vi "WaveformChartGraph-Ver2.vi"() -> ()   [LabVIEW 2019]
panel:
  in  "OK Button":bool
  out "Array":dbl[](array[numeric])
  out "Waveform Graph":dbl[](graph)
  out "Waveform Chart":dbl(graph)
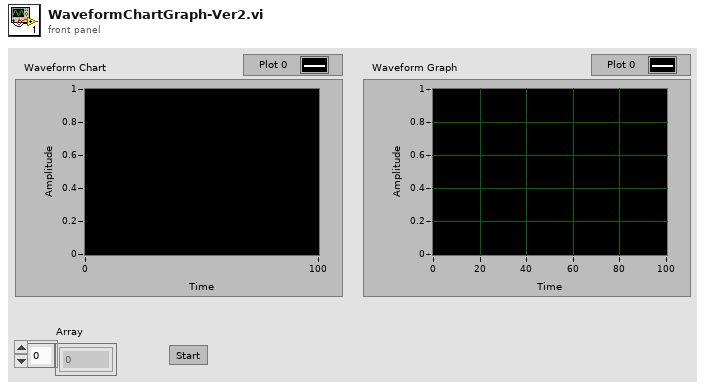
[diagram p1: front panel]
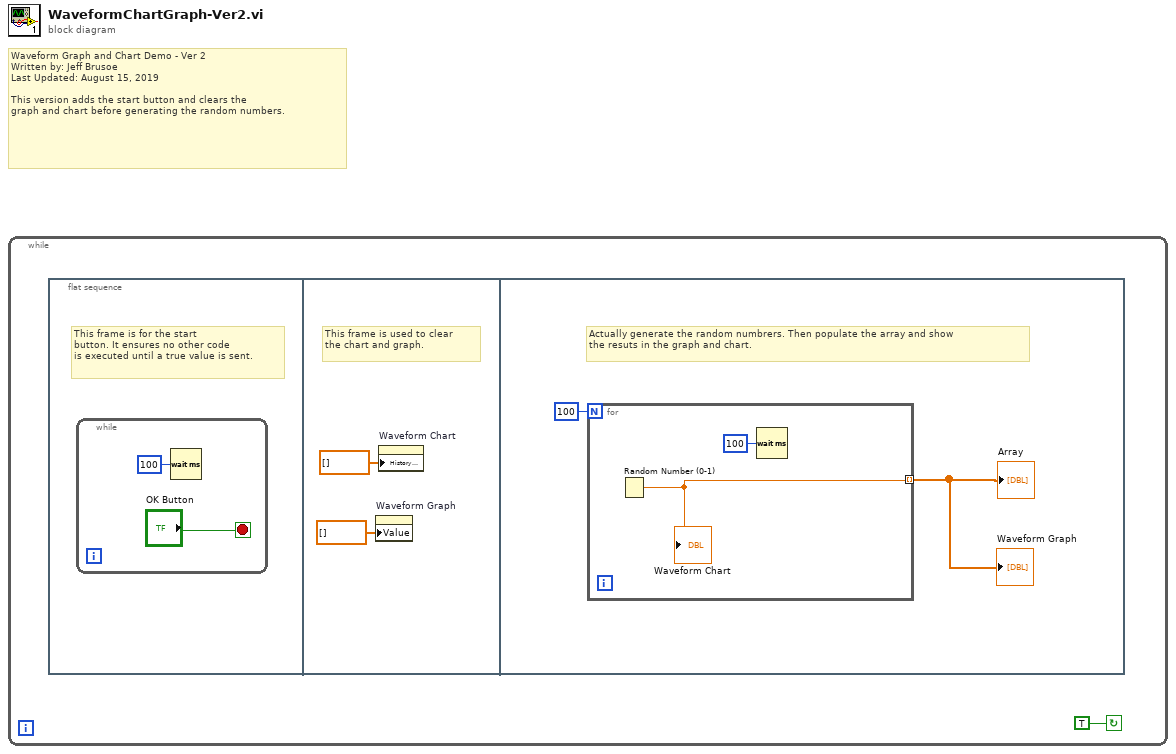
[diagram p0: block diagram]
diagram:
  # "Waveform Graph and Chart Demo - Ver 2\nWritten by: Jeff Brusoe\nLast Updated: August 15, 2019\n\nThis version adds the start button and clears the \ngraph and chart before generating the random numbers."
  n1 = while {
    stop <- TRUE continue-if-true
    n2 = flat-sequence {
      frame #0 {
        # "This frame is for the start\nbutton. It ensures no other code\nis executed until a true value is sent."
        n3 = while {
          stop <- "OK Button" stop-if-true
          n4 = Wait (ms)(milliseconds to wait=u32 100) -> ()  [unwired: 1 out]
        }
      }
      frame #1 {
        # "This frame is used to clear\nthe chart and graph."
        n5 = property on="Waveform Graph" class="WFGraph (strict)"("Value"=dbl[] [] ("Waveform Graph")) -> ()  [unwired: 2 in, 2 out]
        n6 = property on="Waveform Chart" class="WFChart (strict)"("History Data"=dbl[] []) -> ()  [unwired: 2 in, 2 out]
      }
      frame #2 {
        # "Actually generate the random numbrers. Then populate the array and show\nthe resuts in the graph and chart."
        n7 = for {
          N: 100 -> [_]
          tunnel: [w9] -> w7 mode=indexing
          n8 = Random Number (0-1)() -> (number: 0 to 1=w9:dbl)
          "Waveform Chart" <- w9
          n9 = Wait (ms)(milliseconds to wait=u32 100) -> ()  [unwired: 1 out]
        }
        "Waveform Graph" <- w7
        "Array" <- w7
      }
    }
  }
